vi "Read Pressure Servo Valve 1 Setpoint.vi"(11 "IActuatorCylinder in":refnum<class "ILCControlledActuatorCylinder.lvclass">) -> (2 "Pressure Servo Valve 1 Setpoint":dbl[unit], 3 "IActuatorCylinder out":refnum<class "ILCControlledActuatorCylinder.lvclass">)   [LabVIEW 2015, in "ILCControlledActuatorCylinder.lvclass"]
uses:
  ILCControlledActuatorCylinder.lvclass
  ILCControlledActuatorCylinder.lvclass/ILCControlledActuatorCylinder.ctl
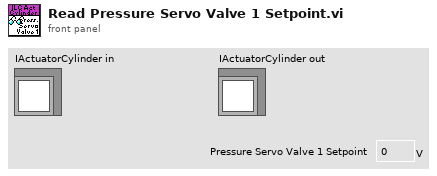
[diagram p1: front panel]
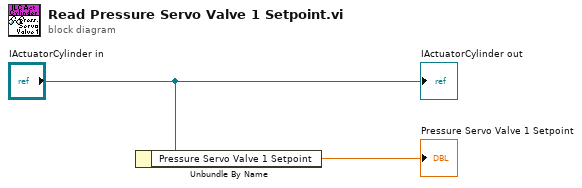
[diagram p0: block diagram]
diagram:
  n1 = Unbundle By Name("IActuatorCylinder in") -> ("Pressure Servo Valve 1 Setpoint"=→"Pressure Servo Valve 1 Setpoint":dbl[unit])
  "IActuatorCylinder out" <- "IActuatorCylinder in"
